vi "LabVIEW Hiss.vi"() -> ()   [LabVIEW 2020]
uses:
  States.ctl
  847b5a13-e703-4616-aa18-4e34a9f91cdc.vi
  <vilib>/Comparison/Equal/Equal Functor/Equal Functor.lvclass
panel:
  out "Potentiometervärde [Ohm]":dbl
  out "Nuvarande tillstånd":variant
  in  "Hissfart [V]":dbl=5.0
  in  "Våning":cluster{"1":bool, "2":bool, "3":bool}
  out "?":cluster{"1":bool, "\n2":bool, "3":bool}
  in  "?":bool
  out "Målvärde [Ohm]":dbl
  out "Våningstolerans [Ohm]":dbl
  out "Våningshöjd [Ohm]":dbl
  in  "Avsluta":bool
  in  "GPIB-addresser":T1={"Funktionsgenerator"="1", "Multimeter"="3", "Nätaggregat"="2"}
  in  "Antal våningar":i32=5
  in  "Tolerans relativt \nvåningshöjd":i32=5
  in  "Potentiometerinställningar":T2
  # "HISSPANEL"
  # "INSTÄLLNINGAR"
  # "FELSÖKNING"
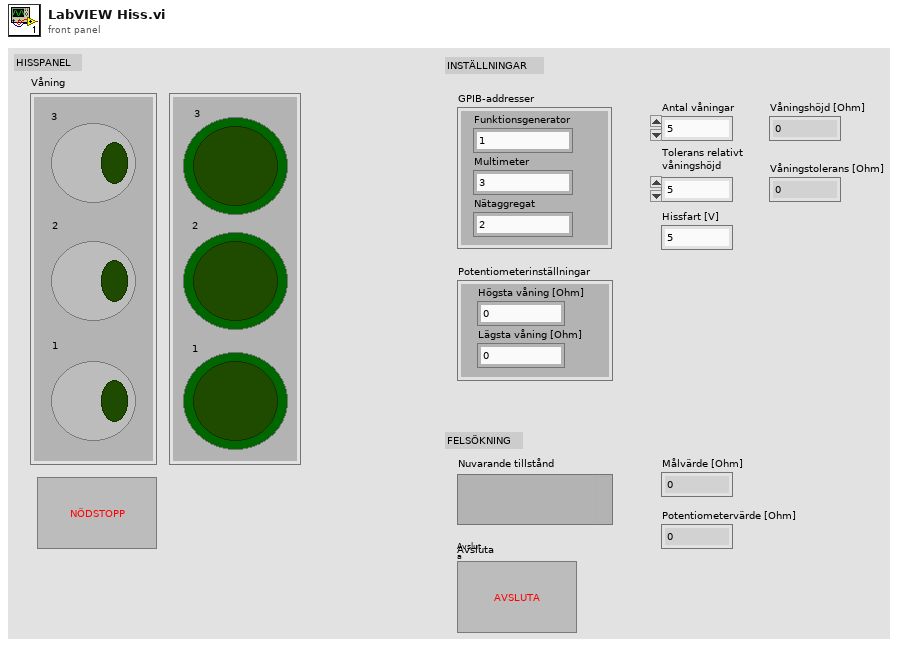
[diagram p1: front panel]
types:
  T1 = cluster{"Funktionsgenerator":string, "Multimeter":string, "Nätaggregat":string}
  T2 = cluster{"Högsta våning [Ohm]":dbl, "Lägsta våning [Ohm]":dbl}
  T3 = cluster{"Våningshöjd":dbl, "Våningstolerans":dbl, "Högsta våning":dbl, "Lägsta våning":dbl, "Hissfart":dbl}
  T4 = typedef "States.ctl" = enum16{"Initialtillstånd", "Kör ner", "Kör upp", "Vänta på input", "Spela ljudfil", "Nödstopp"}
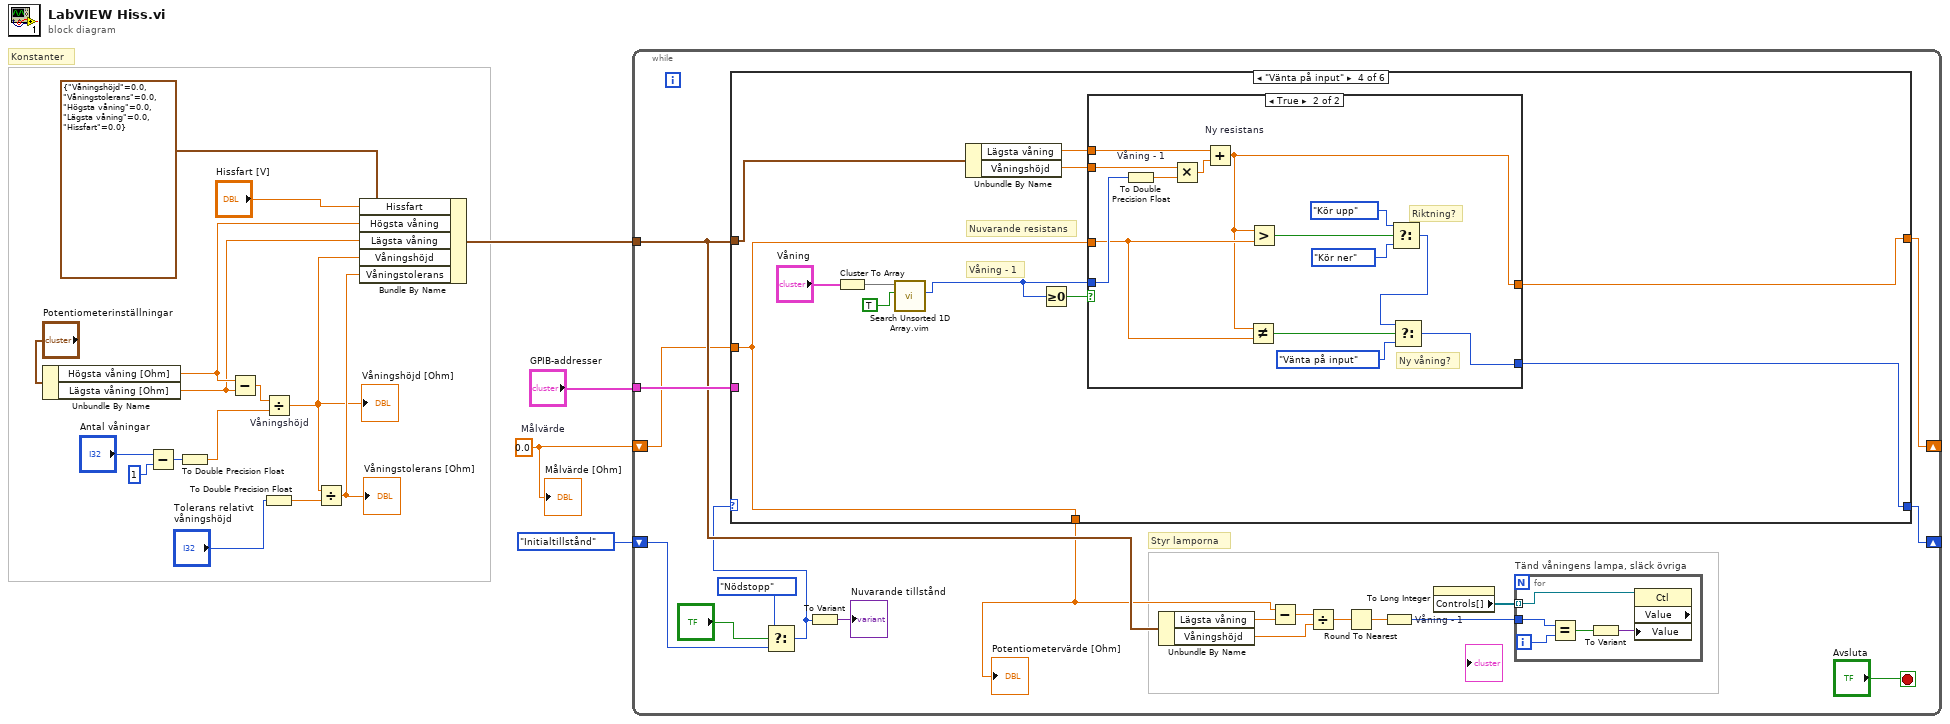
[diagram p0: block diagram]
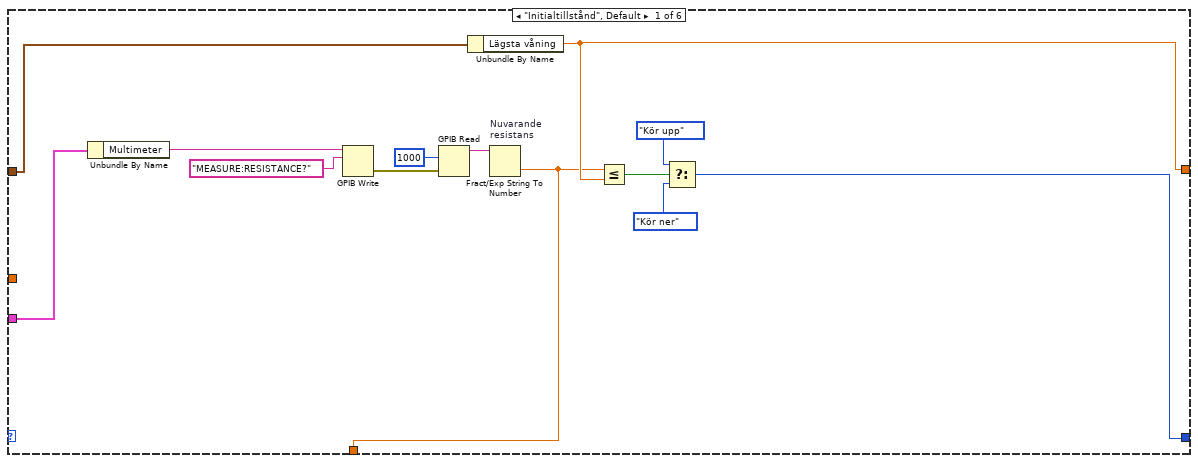
[diagram p2: hidden frame]
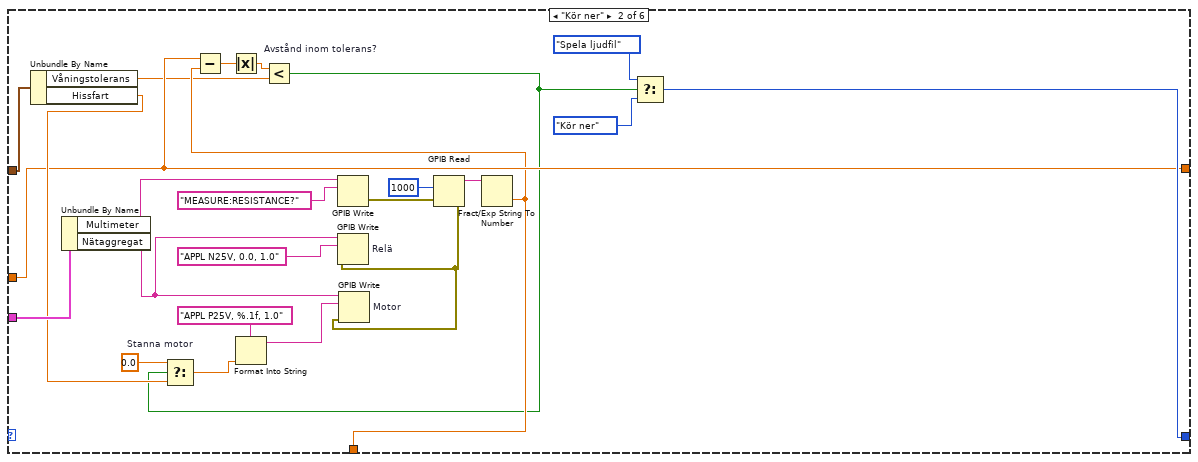
[diagram p3: hidden frame]
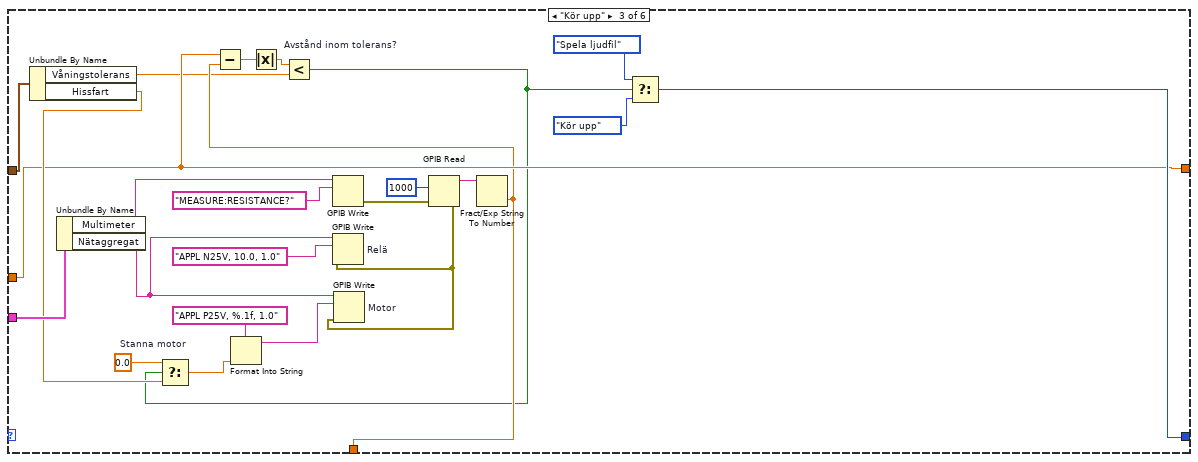
[diagram p4: hidden frame]
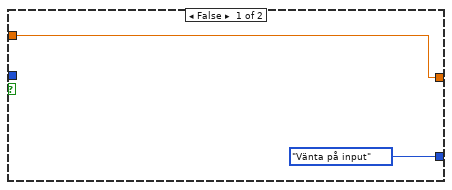
[diagram p5: hidden frame]
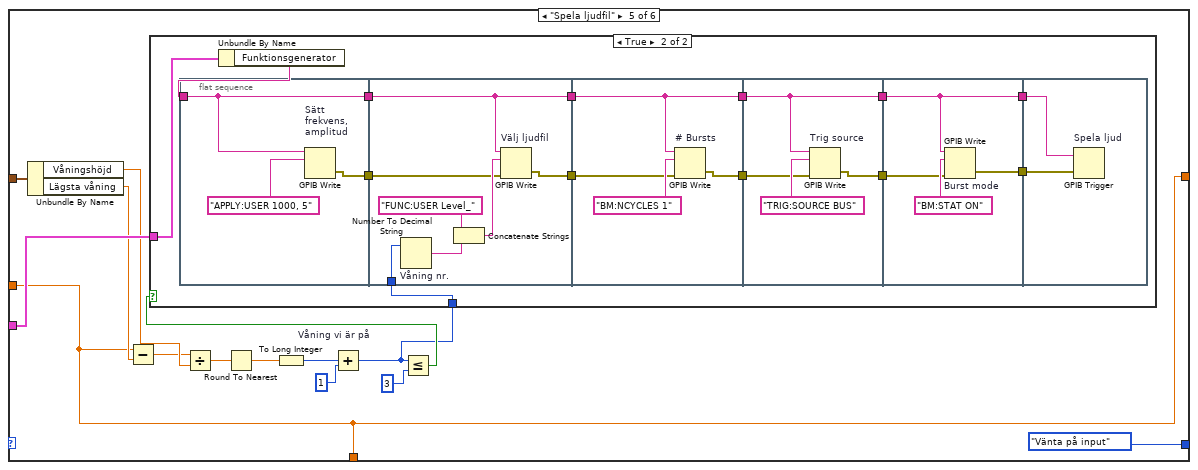
[diagram p6: hidden frame]
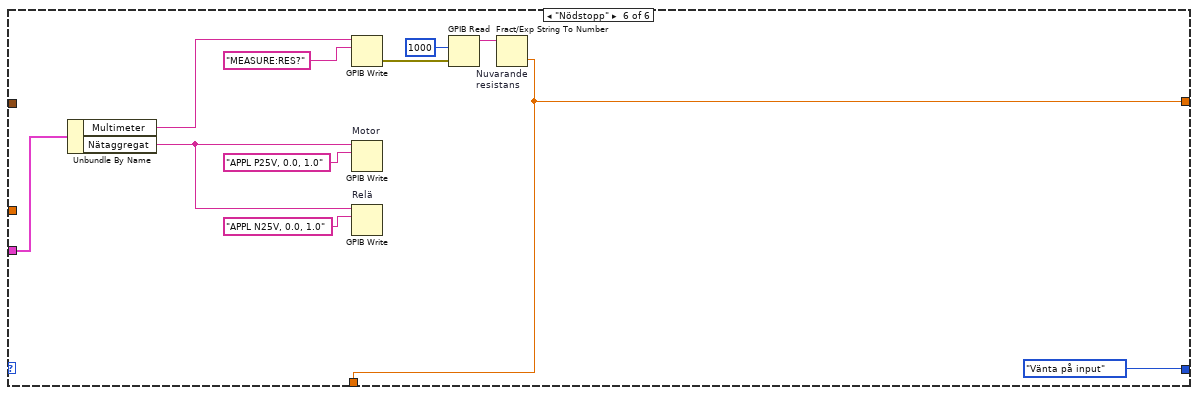
[diagram p8: hidden frame]
diagram:
  w1 = 0.0  # Målvärde
  # "Konstanter"
  n1 = Unbundle By Name("Potentiometerinställningar") -> ("Högsta våning [Ohm]"=w3:dbl, "Lägsta våning [Ohm]"=w2:dbl)
  n2 = Subtract(x="Antal våningar", y=1) -> (x-y=w15:i32)
  n3 = To Double Precision Float(number=w15) -> (double precision float=w14:dbl)
  n4 = Subtract(x=w3, y=w2) -> (x-y=w16:dbl)
  n5 = Divide "Våningshöjd"(x=w16, y=w14) -> (x/y=w4:dbl)
  "Våningshöjd [Ohm]" <- w4
  n6 = To Double Precision Float(number="Tolerans relativt \nvåningshöjd") -> (double precision float=w13:dbl)
  n7 = Divide(x=w4, y=w13) -> (x/y=w5:dbl)
  "Våningstolerans [Ohm]" <- w5
  n8 = Bundle By Name(cluster=T3 {"Våningshöjd"=0.0, "Våningstolerans"=0.0, "Högsta våning"=0.0, "Lägsta våning"=0.0, "Hissfart"=0.0} ("Konstanter"), "Hissfart"="Hissfart [V]", "Högsta våning"=w3, "Lägsta våning"=w2, "Våningshöjd"=w4, "Våningstolerans"=w5) -> (w11:T3)
  n9 = while {
    shift-right: [w33] -> _
    shift-left: States."Initialtillstånd" -> [w36]
    tunnel: "GPIB-addresser" -> [w34]
    shift-right: [w32] -> _
    shift-left: w1 -> [w22]
    tunnel: w11 -> [w27]
    stop <- "Avsluta" stop-if-true
    # "Styr lamporna"
    n10 = Select(t=States."Nödstopp", s="?", f=w36) -> (s? t:f=w21:T4)
    n11 = case shown="\"Vänta på input\"" w21 {
      tunnel: w34 -> [w55 w65 w90 _ w144 w192]
      tunnel: [w46 w64 w89 w110 States."Vänta på input" States."Vänta på input"] -> w33
      tunnel: [w45 w61 w83 w109 w131 w182] -> w32
      tunnel: w27 -> [w44 w66 w91 w113 w143 _]
      tunnel: w22 -> [_ w61 w83 w108 w131 _]
      tunnel: [w43 w60 w82 w108 w131 w182] -> w19
      frame "Initialtillstånd", Default {
        n12 = Unbundle By Name(w55) -> ("Multimeter"=w54:string)
        n13 = GPIB Write(0:w54, 1:"MEASURE:RESISTANCE?") -> (6:w52:errorcluster)  [unwired: 3 in, 1 out]
        n14 = GPIB Read(1:1000, 3:w52) -> (5:w50:string)  [unwired: 3 in, 2 out]
        n15 = Unbundle By Name(w44) -> ("Lägsta våning"=w45:dbl)
        n16 = Fract/Exp String To Number "Nuvarande\nresistans"(string=w50) -> (number=w43:dbl)  [unwired: 3 in, 1 out]
        n17 = Less Or Equal?(x=w43, y=w45) -> (x <= y?=w49:bool)
        n18 = Select(t=States."Kör upp", s=w49, f=States."Kör ner") -> (s? t:f=w46:T4)
      }
      frame "Kör ner" {
        w73 = 0.0  # Stanna motor
        n19 = Unbundle By Name(w66) -> ("Våningstolerans"=w57:dbl, "Hissfart"=w62:dbl)
        n20 = Unbundle By Name(w65) -> ("Multimeter"=w67:string, "Nätaggregat"=w71:string)
        n21 = GPIB Write(0:w67, 1:"MEASURE:RESISTANCE?") -> (6:w78:errorcluster)  [unwired: 3 in, 1 out]
        n22 = GPIB Read(1:1000, 3:w78) -> (5:w76:string, 7:w63:errorcluster)  [unwired: 3 in, 1 out]
        n23 = GPIB Write "Relä"(0:w71, 1:"APPL N25V, 0.0, 1.0", 3:w63) -> ()  [unwired: 2 in, 2 out]
        n24 = Fract/Exp String To Number(string=w76) -> (number=w60:dbl)  [unwired: 3 in, 1 out]
        n25 = Subtract(x=w61, y=w60) -> (x-y=w59:dbl)
        n26 = Absolute Value ("Avstånd")(x=w59) -> (abs(x)=w58:dbl)
        n27 = Less? "Avstånd inom tolerans?"(x=w58, y=w57) -> (x < y?=w56:bool)
        n28 = Select(t=w73, s=w56, f=w62) -> (s? t:f=w72:dbl)
        n29 = Format Into String(format string="APPL P25V, %.1f, 1.0", w72) -> (resulting string=w74:string)  [unwired: 2 in, 1 out]
        n30 = GPIB Write "Motor"(0:w71, 1:w74, 3:w63) -> ()  [unwired: 2 in, 2 out]
        n31 = Select(t=States."Spela ljudfil", s=w56, f=States."Kör ner") -> (s? t:f=w64:T4)
      }
      frame "Kör upp" {
        w97 = 0.0  # Stanna motor
        n32 = Unbundle By Name(w91) -> ("Våningstolerans"=w81:dbl, "Hissfart"=w86:dbl)
        n33 = Unbundle By Name(w90) -> ("Multimeter"=w88:string, "Nätaggregat"=w95:string)
        n34 = GPIB Write(0:w88, 1:"MEASURE:RESISTANCE?") -> (6:w102:errorcluster)  [unwired: 3 in, 1 out]
        n35 = GPIB Read(1:1000, 3:w102) -> (5:w100:string, 7:w87:errorcluster)  [unwired: 3 in, 1 out]
        n36 = GPIB Write "Relä"(0:w95, 1:"APPL N25V, 10.0, 1.0", 3:w87) -> ()  [unwired: 2 in, 2 out]
        n37 = Fract/Exp String To Number(string=w100) -> (number=w82:dbl)  [unwired: 3 in, 1 out]
        n38 = Subtract(x=w83, y=w82) -> (x-y=w85:dbl)
        n39 = Absolute Value ("Avstånd")(x=w85) -> (abs(x)=w84:dbl)
        n40 = Less? "Avstånd inom tolerans?"(x=w84, y=w81) -> (x < y?=w80:bool)
        n41 = Select(t=w97, s=w80, f=w86) -> (s? t:f=w96:dbl)
        n42 = Format Into String(format string="APPL P25V, %.1f, 1.0", w96) -> (resulting string=w98:string)  [unwired: 2 in, 1 out]
        n43 = GPIB Write "Motor"(0:w95, 1:w98, 3:w87) -> ()  [unwired: 2 in, 2 out]
        n44 = Select(t=States."Spela ljudfil", s=w80, f=States."Kör upp") -> (s? t:f=w89:T4)
      }
      frame "Vänta på input" {
        # "Nuvarande resistans"
        # "Våning - 1"
        n45 = Cluster To Array(cluster="Våning") -> (array=w107:bool[])
        n46 = call "Search Unsorted 1D Array.vim"("element"=TRUE, "unsorted 1D array"=w107) -> ("index of element"=w104:i32)  [unwired: 9 in]
        n47 = Unbundle By Name(w113) -> ("Lägsta våning"=w111:dbl, "Våningshöjd"=w112:dbl)
        n48 = Greater Or Equal To 0?(x=w104) -> (x >= 0?=w105:bool)
        n49 = case shown="True" w105 {
          tunnel: w112 -> [_ w130]
          tunnel: w111 -> [_ w128]
          tunnel: [States."Vänta på input" w122] -> w110
          tunnel: w108 -> [w116 w119]
          tunnel: [w116 w117] -> w109
          tunnel: w104 -> [_ w120]
          frame False {
          }
          frame True {
            # "Ny våning?"
            # "Riktning?"
            n50 = To Double Precision Float "Våning - 1"(number=w120) -> (double precision float=w121:dbl)
            n51 = Multiply(x=w130, y=w121) -> (x*y=w129:dbl)
            n52 = Add "Ny resistans"(x=w128, y=w129) -> (x+y=w117:dbl)
            n53 = Not Equal?(x=w117, y=w119) -> (x != y?=w118:bool)
            n54 = Greater?(x=w117, y=w119) -> (0:w127:bool)
            n55 = Select(t=States."Kör upp", s=w127, f=States."Kör ner") -> (s? t:f=w123:T4)
            n56 = Select(t=w123, s=w118, f=States."Vänta på input") -> (s? t:f=w122:T4)
          }
        }
      }
      frame "Spela ljudfil" {
        n57 = Unbundle By Name(w143) -> ("Våningshöjd"=w141:dbl, "Lägsta våning"=w142:dbl)
        n58 = Subtract(x=w131, y=w142) -> (x-y=w140:dbl)
        n59 = Divide(x=w140, y=w141) -> (x/y=w139:dbl)
        n60 = Round To Nearest(number=w139) -> (nearest integer value=w138:dbl)
        n61 = To Long Integer(number=w138) -> (32bit integer=w137:i32)
        n62 = Add "Våning vi är på"(x=w137, y=1) -> (x+y=w132:i32)
        n63 = Less Or Equal?(x=w132, y=3) -> (x <= y?=w134:bool)
        n64 = case shown="True" w134 {
          tunnel: w144 -> [_ w157]
          tunnel: w132 -> [_ w150]
          frame False {
          }
          frame True {
            n65 = flat-sequence {
              tunnel: w156 -> [w159]
              tunnel: [w159] -> w155
              tunnel: [w158] -> w149
              tunnel: w155 -> [w163]
              tunnel: w150 -> [w167]
              tunnel: [w163] -> w154
              tunnel: w149 -> [w162]
              tunnel: [w161] -> w148
              tunnel: w154 -> [w171]
              tunnel: [w171] -> w153
              tunnel: w148 -> [w169]
              tunnel: [w168] -> w147
              tunnel: w153 -> [w175]
              tunnel: [w175] -> w152
              tunnel: w147 -> [w173]
              tunnel: [w172] -> w146
              tunnel: w152 -> [w179]
              tunnel: [w179] -> w151
              tunnel: w146 -> [w177]
              tunnel: [w176] -> w145
              tunnel: w151 -> [w181]
              tunnel: w145 -> [w180]
              frame #0 {
                n66 = GPIB Write "Sätt\nfrekvens,\namplitud"(0:w159, 1:"APPLY:USER 1000, 5") -> (6:w158:errorcluster)  [unwired: 3 in, 1 out]
              }
              frame #1 {
                n67 = Number To Decimal String "Våning nr."(number=w167) -> (decimal integer string=w165:string)  [unwired: 1 in]
                n68 = Concatenate Strings("FUNC:USER Level_", w165) -> (w164:string)
                n69 = GPIB Write "Välj ljudfil"(0:w163, 1:w164, 3:w162) -> (6:w161:errorcluster)  [unwired: 2 in, 1 out]
              }
              frame #2 {
                n70 = GPIB Write "# Bursts"(0:w171, 1:"BM:NCYCLES 1", 3:w169) -> (6:w168:errorcluster)  [unwired: 2 in, 1 out]
              }
              frame #3 {
                n71 = GPIB Write "Trig source"(0:w175, 1:"TRIG:SOURCE BUS", 3:w173) -> (6:w172:errorcluster)  [unwired: 2 in, 1 out]
              }
              frame #4 {
                n72 = GPIB Write "Burst mode"(0:w179, 1:"BM:STAT ON", 3:w177) -> (6:w176:errorcluster)  [unwired: 2 in, 1 out]
              }
              frame #5 {
                n73 = GPIB Trigger "Spela ljud"(2:w180, 3:w181) -> ()  [unwired: 2 out]
              }
            }
            n74 = Unbundle By Name(w157) -> ("Funktionsgenerator"=w156:string)
          }
        }
      }
      frame "Nödstopp" {
        n75 = Unbundle By Name(w192) -> ("Multimeter"=w183:string, "Nätaggregat"=w189:string)
        n76 = GPIB Write(0:w183, 1:"MEASURE:RES?") -> (6:w187:errorcluster)  [unwired: 3 in, 1 out]
        n77 = GPIB Write "Motor"(0:w189, 1:"APPL P25V, 0.0, 1.0") -> ()  [unwired: 3 in, 2 out]
        n78 = GPIB Write "Relä"(0:w189, 1:"APPL N25V, 0.0, 1.0") -> ()  [unwired: 3 in, 2 out]
        n79 = GPIB Read(1:1000, 3:w187) -> (5:w185:string)  [unwired: 3 in, 2 out]
        n80 = Fract/Exp String To Number "Nuvarande\nresistans"(string=w185) -> (number=w182:dbl)  [unwired: 3 in, 1 out]
      }
    }
    "Potentiometervärde [Ohm]" <- w19
    n81 = To Variant(anything=w21) -> (Variant=→"Nuvarande tillstånd":variant)
    n82 = Unbundle By Name(w27) -> ("Lägsta våning"=w26:dbl, "Våningshöjd"=w25:dbl)
    n83 = Subtract(x=w19, y=w26) -> (x-y=w30:dbl)
    n84 = Divide(x=w30, y=w25) -> (x/y=w29:dbl)
    n85 = Round To Nearest(number=w29) -> (nearest integer value=w28:dbl)
    n86 = To Long Integer "Våning - 1"(number=w28) -> (32bit integer=w24:i32)
    n87 = property class="Clust (strict)"() -> ("Controls[]"=w23:refnum<vi>[])  [unwired: 2 in, 2 out]
    n88 = for "Tänd våningens lampa, släck övriga" {
      tunnel: w24 -> [w41]
      tunnel: w23 -> [w42] mode=indexing
      i -> [w40]
      n89 = Equal?(x=w41, y=w40) -> (x = y?=w38:bool)
      n90 = To Variant(anything=w38) -> (Variant=w39:variant)
      n91 = property class="Ctl" props=["Value", "Value"](reference=w42, "Value"=w39) -> ()  [unwired: 1 in, 3 out]
    }
  }
  "Målvärde [Ohm]" <- w1
